vi "Micro-PL v10.0.0.vi"() -> ()   [LabVIEW 2010]
uses:
  drivers/Oxford ITC/ITCAPPS.LLB/ITCSetup.ctl
  drivers/Oxford ITC/ITCSUBS.LLB/ITCIO.ctl
  drivers/Oxford ITC/BUSGEN.LLB/OxfordAddress.ctl
  drivers/Oxford ITC/ITCSUBS.LLB/ITCVersion.ctl
  subvi/ESA-C/TypeDefs/ESA-C Live Controls.ctl
  subvi/ESA-C/TypeDefs/ESA-C Current Values.ctl
  subvi/ESA-C/TypeDefs/ESA-C Connection Settings.ctl
  subvi/ESA-C/TypeDefs/ESA-C Set Positions.ctl
  subvi/ITC503/TypeDefs/ITC503 Settings.ctl
  subvi/ITC503/TypeDefs/ITC503 Current Values.ctl
  subvi/iHR550/TypeDefs/iHR Current Values.ctl
  subvi/iHR550/TypeDefs/iHR Settings.ctl
  subvi/Mapping/TypeDefs/Mapping Spectra Params.ctl
  <vilib>/Utility/miscctls.llb/LVPointTypeDef.ctl
  drivers/Horiba Spectrum One 3000V/Lib/CCD_command.llb/Comm Params.ctl
panel:
  out "Int. Time Temp":dbl
  out "Wavelengths (nm)":dbl[](array[numeric])
  out "Measurement Running":bool
  out "ITC503s Running":bool
  out "Drive Running":bool
  out "CCD3500V Running":bool
  out "iHR550 Running":bool
  in  "Exit":bool
  out "iHR550 Status":bool
  out "Drive Status":bool
  out "CCD3500V Status":bool
  out "ITC503 Status":bool
  in  "CCD3500V Connection":T1={"Comm Interface"=1, "BUS"=0, "Address"=5, "Com Port"=0}
  out "Video Running":bool
  out "iHR550 RefNum":refnum<k7> caption="Mono RefNum out"
  out "ITC Setup":T2={"Description"="", "IO Info"={"Address"={"Com Port"=1, "ISOBUS Address"=1, "GPIB Address"=24, "Communication"=enum."ISOBUS"}, "Version"=enum."ITC503", "Ch 1 dec places"=1, "Ch 2 dec places"=1, "Ch 3 dec places"=1, "Ch1 Name"="", "Ch2 Name"="", "Ch3 Name"=""}}
  in  "Register":T6(tab)
  in  "iHR550 Force Init":bool=TRUE
  in  "iHR550 Connect":bool
  in  "iHR550 ID":string(combo)="iHR550" caption="Monochromator ID"
  out "ITC503 Current Values":T7 {"ITC503 Gradient" format="%.2f"; "ITC503 Setpoint" min=-273.0 max=300000.0 step=0.0001 format="%.1f"; "ITC503 I" format="%_1f"; "ITC503 P" format="%_1f"; "ITC503 Temperature" min=0.0 max=1645.0 step=1e-05 format="%.2f"; "ITC503 Heater" min=0.0 max=100.0 step=0.01 scale=0.0..100.0}
  in  "ITC503 Settings":T8={"ITC503 Set Setpoint"=0.0, "ITC503 Set Auto Heater"=TRUE, "ITC503 Set Auto PID"=TRUE, "P"=0.0, "I"=0.0, "D"=0.0} {"D" min=0.0 max=100.0 step=0.1 format="%.1f"; "I" min=0.0 max=100.0 step=0.1 format="%.1f"; "P" min=0.0 max=100.0 step=0.1 format="%.1f"; "ITC503 Set Setpoint" min=-273.0 max=300000.0 step=0.1 format="%.1f"}
  in  "ITC503 Configure":bool
  in  "ITC503 Connect":bool
  in  "ITC503 Selector":u16(ring) caption="Select Device" items=["ITC503s"]
  out "Drive Current Values":T9 {"Position"."Drive Z Position" min=-273.0 max=300000.0 step=0.0001 format="%.1f"; "Position"."Drive Y Position" min=-273.0 max=300000.0 step=0.0001 format="%.1f"; "Position"."Drive X Position" min=-273.0 max=300000.0 step=0.0001 format="%.1f"; "Voltages"."Drive Z Voltage" min=-273.0 max=300000.0 step=0.0001 format="%.1f"; "Voltages"."Drive Y Voltage" min=-273.0 max=300000.0 step=0.0001 format="%.1f"; "Voltages"."Drive X Voltage" min=-273.0 max=300000.0 step=0.0001 format="%.1f"}
  in  "Drive Connection":T10={"Objective GPIB-Port"=4, "Stage GPIB-Port"=4, "Drive Selector"=0, "Drive Velocity (V/s)"=5.0} {"Drive Velocity (V/s)" min=10.0 max=160.0 step=0.1 format="%.1f"; "Drive Selector" items=["Obj.", "Stage"]; "Stage GPIB-Port" min=1 max=20 step=1 format="%#.0f"; "Objective GPIB-Port" min=1 max=20 step=1 format="%#.0f"}
  in  "Drive Connect":bool
  out "CCD3500 Temperature":dbl caption="Temp. (°C)" min=10.0 max=160.0 step=0.1 format="%.1f"
  in  "CCD3500V GPIB-Port":i32=5 caption="GPIB-Port" min=1 max=20 step=1 format="%#.0f"
  in  "CCD3500V Connect":bool
  in  "CCD3000 Current Rep.":string="0/0"
  in  "Video Show":bool
  in  "Drive GoTo":bool caption="Objective Move Abs."
  in  "Drive New Positions":T11 {"Drive X Set" min=10.0 max=160.0 step=0.1 format="%.1f"; "Drive Z Set" min=10.0 max=160.0 step=0.1 format="%.1f"; "Drive Y Set" min=10.0 max=160.0 step=0.1 format="%.1f"}
  in  "Spectrum Autosave":bool=TRUE caption="iHR550 Force Init"
  in  "CCD3500 Preview":bool
  in  "CCD3500 Acquire":bool
  in  "Spectra Settings":T12={"Integration Time"=1.0, "Repetitions"=1, "Mapping Spectra"=TRUE} caption="Mapping Spectra Settings" {"Repetitions" min=1 max=100 step=1; "Integration Time" min=0.1 max=6000.0 step=0.1 format="%.1f"}
  in  "Spectrum Save":bool
  out "Spectrum":cluster{dbl[], dbl[]}(graph)
  in  "Mapping Start":bool
  in  "iHR550 Configure":bool
  in  "iHR Settings":T13={"iHR550 Set Exit Mirror"=2, "iHR550 Set Side Exit"=0.0, "iHR550 Set Front Entrance"=0.0, "iHR550 Set Wavelength"=897.9988, "iHR550 Set Grating"=0, "iHR550 Set Grating Switch"=FALSE, "iHR550 Set Wavelength Switch"=FALSE, "iHR550 Set Mirror Switch"=FALSE, "iHR550 Set Slits Switch"=FALSE} {"iHR550 Set Grating" items=["1800"=1, "600"=2, "150"=3]; "iHR550 Set Wavelength" min=0.0 max=1500.0 step=1.0; "iHR550 Set Side Exit" min=0.0 max=2000.0 step=1.0; "iHR550 Set Exit Mirror" items=["Front"=2, "Side"=3]}
  out "iHR Current Values":T14={"iHR 550 Front Entrance"=0.0, "iHR550 Side Exit"=0.0, "iHR550 Wavelength"=897.9988, "iHR550 Exit Mirror"=2, "iHR550 Grating"="1", "Grating Index"=1} {"iHR550 Exit Mirror" items=["EntranceMirror", "ExitMirror", "Front", "Side"]}
  out "Drive Live Current Values":T9 {"Position"."Drive Z Position" min=-273.0 max=300000.0 step=0.0001 format="%.1f"; "Position"."Drive Y Position" min=-273.0 max=300000.0 step=0.0001 format="%.1f"; "Position"."Drive X Position" min=-273.0 max=300000.0 step=0.0001 format="%.1f"; "Voltages"."Drive Z Voltage" min=-273.0 max=300000.0 step=0.0001 format="%.1f"; "Voltages"."Drive Y Voltage" min=-273.0 max=300000.0 step=0.0001 format="%.1f"; "Voltages"."Drive X Voltage" min=-273.0 max=300000.0 step=0.0001 format="%.1f"}
  in  "Drive Live Controls":T15={"Snapshot"=FALSE, "Move Step"=1.0, "Move Home"=FALSE, "Move Down"=FALSE, "Move Up"=FALSE, "Move Left"=FALSE, "Move Right"=FALSE, "Move Out"=FALSE, "Move In"=FALSE} {"Move Step" min=0.0 max=30.0 step=0.1 format="%.1f"}
  # "Correlation Setup"
  # "Active"
  # "Active"
  # "ITC"
  # "iHR"
  # "Drive"
  # "CCD"
  # "Status"
  # "CCD"
  # "ITC"
  # "iHR"
  # "Drive"
  # "Monochromator"
  # "Cryostat"
  # "Drives"
  # "CCD-Camera"
  # "Drive Control"
  # "CCD"
  # "Spectrum"
  # "Mapping"
  # "Launch the Spectral Mapping VI and Raman Tool Set 2.0 in a new window."
  # "Monochromator"
  # "XY"
  # "Z"
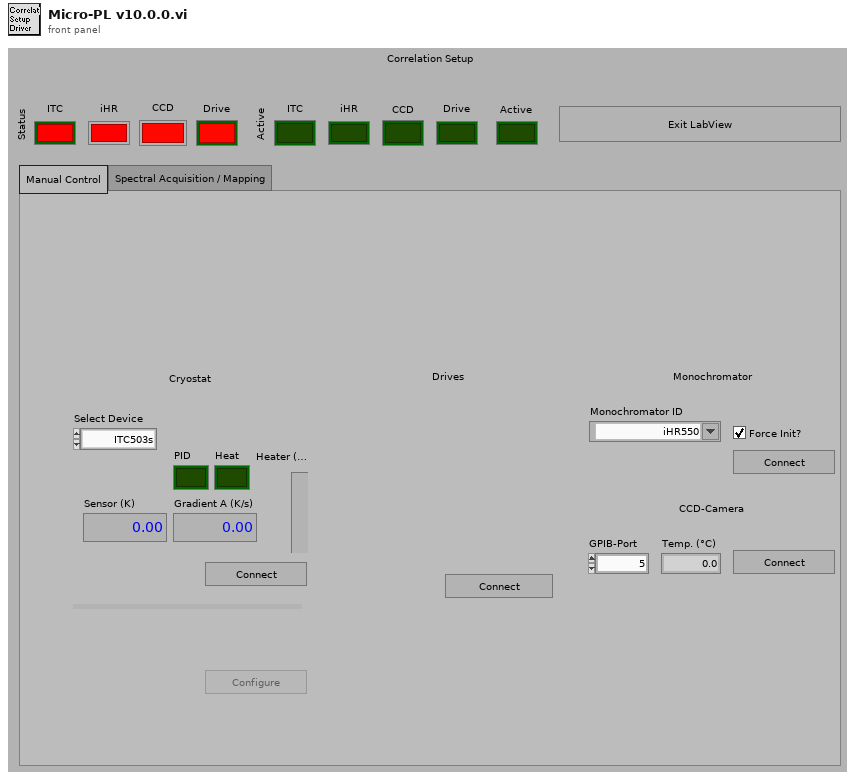
[diagram p1: front panel]
types:
  T1 = cluster{"Comm Interface":u16, "BUS":i16, "Address":i16, "Com Port":i32}
  T2 = typedef "ITCSetup.ctl" = cluster{"Description":string, "IO Info":T3}
  T3 = typedef "ITCIO.ctl" = cluster{"Address":T4, "Version":T5, "Ch 1 dec places":i16, "Ch 2 dec places":i16, "Ch 3 dec places":i16, "Ch1 Name":string, "Ch2 Name":string, "Ch3 Name":string}
  T4 = typedef "OxfordAddress.ctl" = cluster{"Com Port":i32, "ISOBUS Address":i32, "GPIB Address":i16, "Communication":enum16{"RS232", "ISOBUS", "GPIB", "Gateway"}}
  T5 = typedef "ITCVersion.ctl" = enum16{"ITC502", "ITC503", "ITC601"}
  T6 = enum32{"Manual Control", "Spectral Acquisition / Mapping"}
  T7 = typedef "ITC503 Current Values.ctl" = cluster{"ITC503 Heater":dbl, "ITC503 Temperature":dbl, "ITC503 P":dbl, "ITC503 I":dbl, "ITC503 D":dbl, "ITC503 Setpoint":dbl, "ITC503 Gradient":dbl, "ITC503 Heater Auto":bool, "ITC503 PID Auto":bool}
  T8 = typedef "ITC503 Settings.ctl" = cluster{"ITC503 Set Setpoint":dbl, "ITC503 Set Auto Heater":bool, "ITC503 Set Auto PID":bool, "P":dbl, "I":dbl, "D":dbl}
  T9 = typedef "ESA-C Current Values.ctl" = cluster{"Voltages":cluster{"Drive X Voltage":dbl, "Drive Y Voltage":dbl, "Drive Z Voltage":dbl}, "Position":cluster{"Drive X Position":dbl, "Drive Y Position":dbl, "Drive Z Position":dbl}}
  T10 = typedef "ESA-C Connection Settings.ctl" = cluster{"Objective GPIB-Port":i32, "Stage GPIB-Port":i32, "Drive Selector":u16, "Drive Velocity (V/s)":dbl}
  T11 = typedef "ESA-C Set Positions.ctl" = cluster{"Drive X Set":dbl, "Drive Y Set":dbl, "Drive Z Set":dbl}
  T12 = typedef "Mapping Spectra Params.ctl" = cluster{"Integration Time":dbl, "Repetitions":u16, "Mapping Spectra":bool}
  T13 = typedef "iHR Settings.ctl" = cluster{"iHR550 Set Exit Mirror":u16, "iHR550 Set Side Exit":dbl, "iHR550 Set Front Entrance":dbl, "iHR550 Set Wavelength":dbl, "iHR550 Set Grating":u16, "iHR550 Set Grating Switch":bool, "iHR550 Set Wavelength Switch":bool, "iHR550 Set Mirror Switch":bool, "iHR550 Set Slits Switch":bool}
  T14 = typedef "iHR Current Values.ctl" = cluster{"iHR 550 Front Entrance":dbl, "iHR550 Side Exit":dbl, "iHR550 Wavelength":dbl, "iHR550 Exit Mirror":i32, "iHR550 Grating":string, "Grating Index":i32}
  T15 = typedef "ESA-C Live Controls.ctl" = cluster{"Snapshot":bool, "Move Step":dbl, "Move Home":bool, "Move Down":bool, "Move Up":bool, "Move Left":bool, "Move Right":bool, "Move Out":bool, "Move In":bool}
  T16 = typedef "LVPointTypeDef.ctl" = cluster{"Horizontal":i16, "Vertical":i16}
  T17 = enum16{"CCD Temperature Z345", "CCD Temperature Z308", "CCD Gain"}
  T18 = enum8{"Enabled", "Disabled", "Disabled and Grayed Out"}
  T19 = typedef "Comm Params.ctl" = cluster{"Comm Interface":u16, "BUS":i16, "Address":i16, "Com Port":i32}
  T20 = cluster{"CCD3000 Connection":T19, "Drive Connection Settings":T10, "ITC503 Current Values":T7, "Wavelengths (nm)":dbl[], "Drive Current Values":T9, "iHR Current Values":T14, "Spectra Settings":T12, "CCD3500 Temperature":dbl}
  T21 = cluster{"Intensities":dbl[], "Wavelengths":dbl[]}
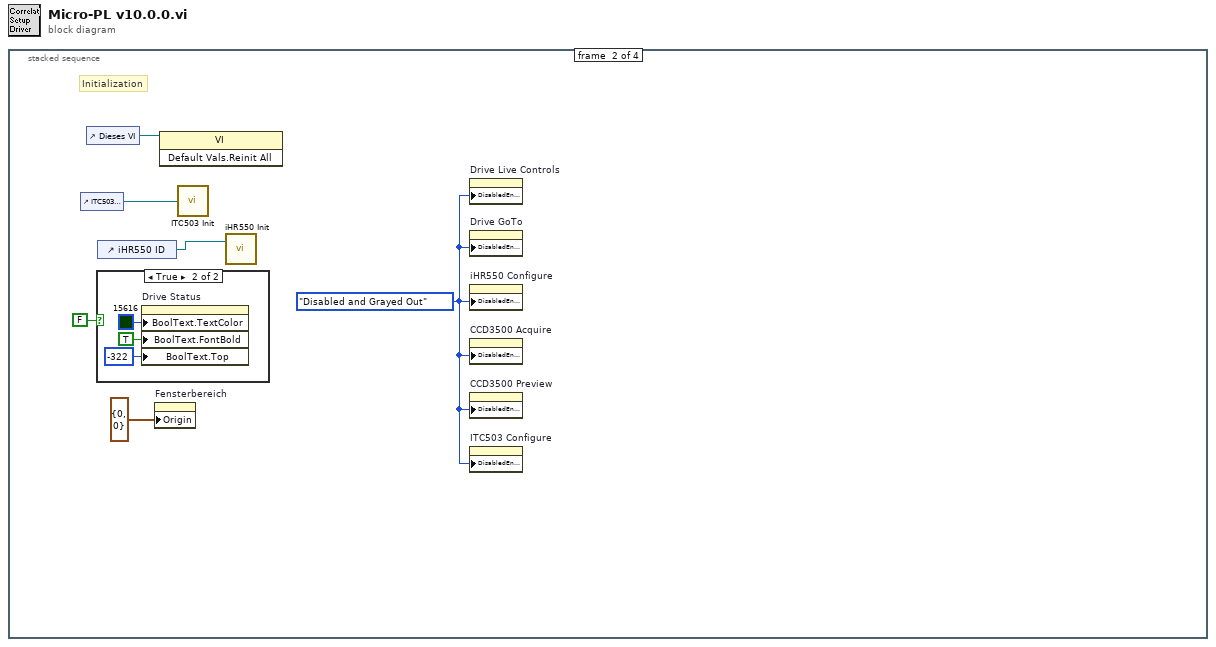
[diagram p0: block diagram]
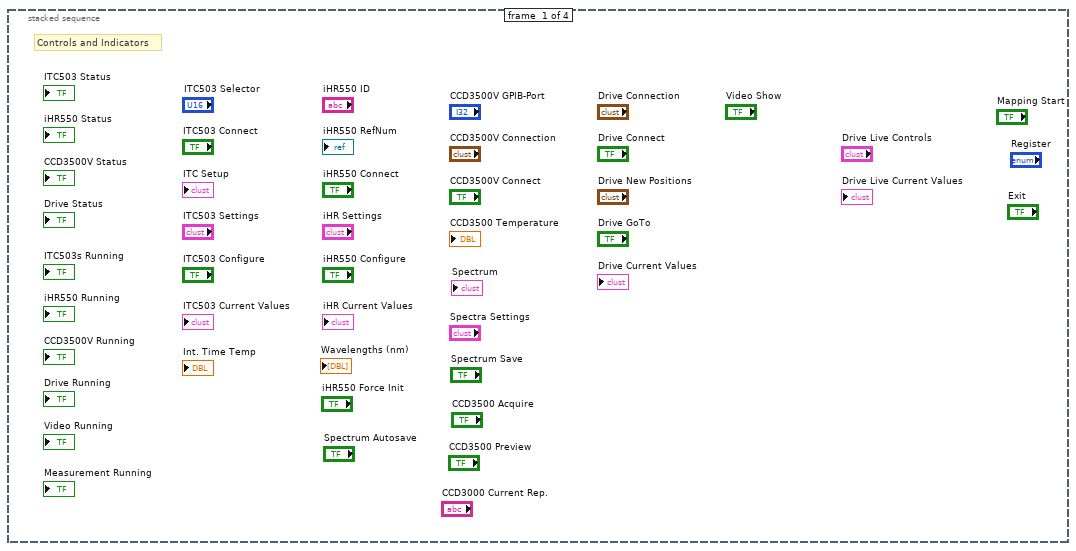
[diagram p2: hidden frame]
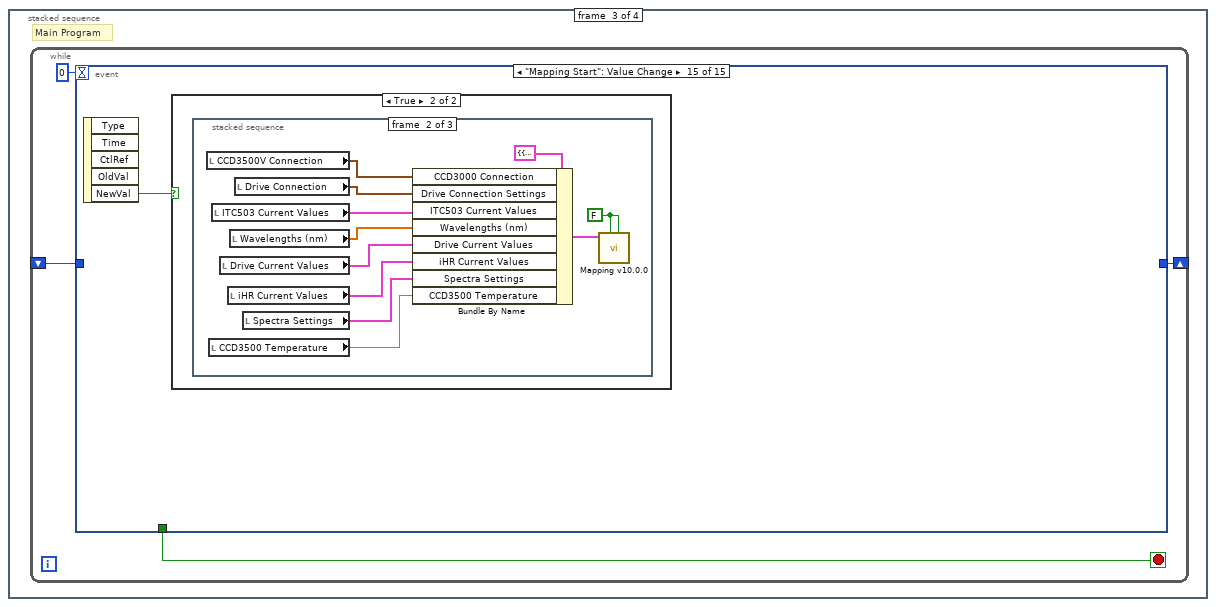
[diagram p4: hidden frame]
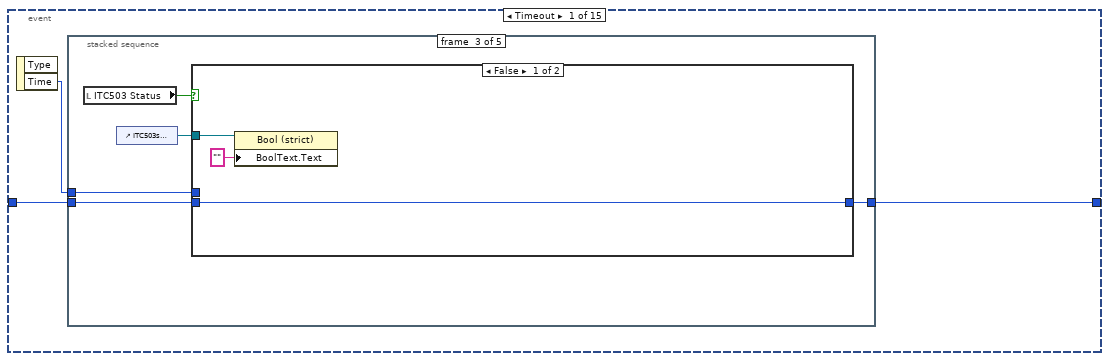
[diagram p5: hidden frame]
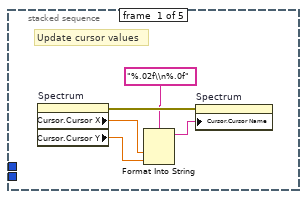
[diagram p6: hidden frame]
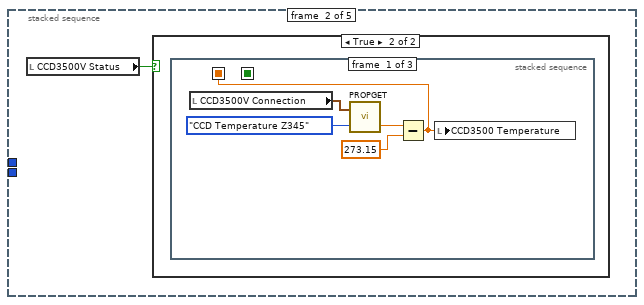
[diagram p7: hidden frame]
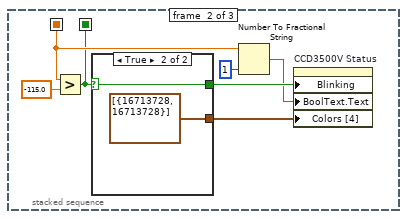
[diagram p9: hidden frame]
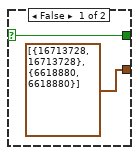
[diagram p10: hidden frame]
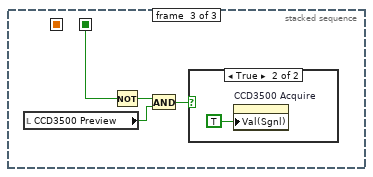
[diagram p11: hidden frame]
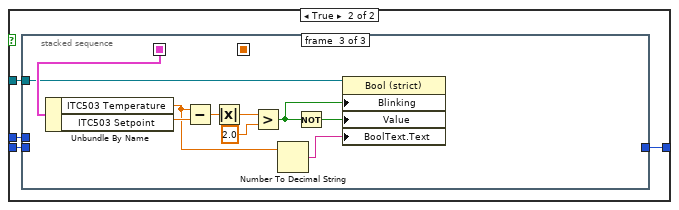
[diagram p13: hidden frame]
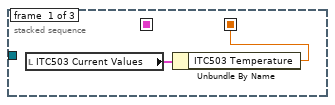
[diagram p14: hidden frame]
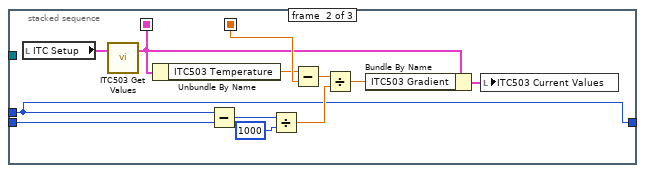
[diagram p15: hidden frame]
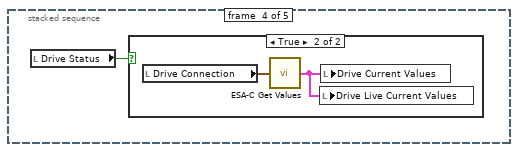
[diagram p16: hidden frame]
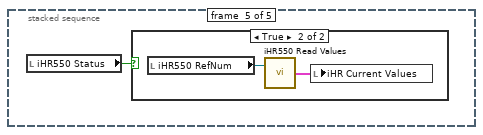
[diagram p18: hidden frame]
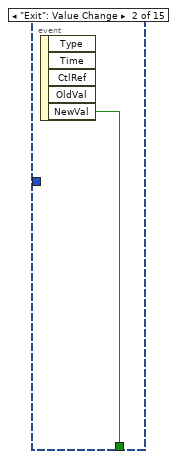
[diagram p20: hidden frame]
diagram:
  n1 = stacked-sequence {
    frame #0 {
      # "Controls and Indicators"
    }
    frame #1 {
      w1 = T18."Disabled and Grayed Out" ("Deaktiviert")
      # "Initialization"
      n2 = control-ref of="ITC503 Selector"() -> (w6:refnum<vi>)
      n3 = control-ref of="Dieses VI"() -> (w5:refnum<vi>)
      n4 = case shown="True" FALSE {
        frame False {
        }
        frame True {
          n5 = property on="Drive Status" class="Bool (strict)"("BoolText.TextColor"=u32 15616, "BoolText.FontBold"=TRUE ("Boolescher Text.Schriftart:Fett"), "BoolText.Top"=-322 ("Boolescher Text.Position:Oben")) -> ()  [unwired: 2 in, 2 out]
        }
      }
      n6 = control-ref of="iHR550 ID"() -> (w4:refnum<vi>)
      n7 = property on="Fensterbereich" class="Pane"("Origin"=T16 {"Horizontal"=0, "Vertical"=0}) -> ()  [unwired: 2 in, 2 out]
      n8 = invoke class="VI" method="Default Vals.Reinit All"(reference=w5) -> ()  [unwired: 2 in, 3 out]
      n9 = call "ITC503 Init.vi"("ITC Selector"=w6) -> ()  [unwired: 1 in]
      n10 = call "iHR550 Init.vi"("Mono ID"=w4) -> ()  [unwired: 2 in]
      n11 = property on="Drive Live Controls" class="Clust (strict)"("DisabledEnum"=w1) -> ()  [unwired: 2 in, 2 out]
      n12 = property on="Drive GoTo" class="Bool (strict)"("DisabledEnum"=w1) -> ()  [unwired: 2 in, 2 out]
      n13 = property on="iHR550 Configure" class="Bool (strict)"("DisabledEnum"=w1) -> ()  [unwired: 2 in, 2 out]
      n14 = property on="CCD3500 Acquire" class="Bool (strict)"("DisabledEnum"=w1) -> ()  [unwired: 2 in, 2 out]
      n15 = property on="CCD3500 Preview" class="Bool (strict)"("DisabledEnum"=w1) -> ()  [unwired: 2 in, 2 out]
      n16 = property on="ITC503 Configure" class="Bool (strict)"("DisabledEnum"=w1) -> ()  [unwired: 2 in, 2 out]
    }
    frame #2 {
      # "Main Program"
      n17 = while "Main-Program" {
        shift-right: [w11] -> _
        shift-left: _ -> [w10]
        stop <- w13 stop-if-true
        n18 = event shown="[14] \"Mapping Start\": Value Change" {
          selector: _ -> [_ _ _ _ _ _ _ _ _ _ _ _ _ _ _]
          dyn-events: _ -> [_ _ _ _ _ _ _ _ _ _ _ _ _ _ _]
          timeout: 0 -> [_ _ _ _ _ _ _ _ _ _ _ _ _ _ _]
          tunnel: [_ w86 _ _ _ _ _ _ _ _ _ _ _ _ _] -> w13
          tunnel: w10 -> [w15 _ _ _ _ _ _ _ _ _ _ _ _ _ _]
          tunnel: [w14 _ _ _ _ _ _ _ _ _ _ _ _ _ _] -> w11
          event Timeout {
            n19 = event-data() -> ("Time"=w16:u32)  [unwired: 1 in, 1 out]
            n20 = stacked-sequence {
              tunnel: w16 -> [_ _ w47 _ _]
              tunnel: w15 -> [_ _ w46 _ _]
              tunnel: [_ _ w45 _ _] -> w14
              frame #0 {
                # "Update cursor values"
                n21 = property on="Spectrum" class="XYGraph (strict)"() -> (error out=w21:errorcluster, "Cursor.Cursor X"=w20:dbl, "Cursor.Cursor Y"=w19:dbl)  [unwired: 2 in, 1 out]
                n22 = Format Into String(format string="%.02f\\n%.0f", w20, w19) -> (resulting string=w17:string)  [unwired: 2 in, 1 out]
                n23 = property on="Spectrum" class="XYGraph (strict)"(error in=w21, "Cursor.Cursor Name"=w17) -> ()  [unwired: 1 in, 2 out]
              }
              frame #1 {
                n24 = local read "CCD3500V Status"() -> (w22:bool)
                n25 = case shown="True" w22 {
                  frame False {
                  }
                  frame True {
                    n26 = stacked-sequence {
                      seq-local: [w23 _ _] -> [_ w32 _]
                      seq-local: [_ w28 _] -> [_ _ w42]
                      frame #0 {
                        n27 = local read "CCD3500V Connection"() -> (w27:T1)
                        n28 = call "PROPGET.VI"("CCD Prop ID"=T17."CCD Temperature Z345", "Comm Params"=w27) -> ("Output Param"=w25:dbl)  [unwired: 1 out]
                        n29 = Subtract(x=w25, y=273.15) -> (x-y=w23:dbl)
                        n30 = local write "CCD3500 Temperature"(w23) -> ()
                      }
                      frame #1 {
                        n31 = Greater?(x=w32, y=-115.0) -> (0:w28:bool)
                        n32 = case shown="True" w28 {
                          selector: w28 -> [w36 w38]
                          tunnel: [cluster{u32, u32}[] [{16713728, 16713728}, {6618880, 6618880}] ("Farben [4]") cluster{u32, u32}[] [{16713728, 16713728}] ("Farben [4]")] -> w29
                          tunnel: [w36 w38] -> w31
                          frame False {
                          }
                          frame True {
                          }
                        }
                        n33 = Number To Fractional String(number=w32, precision (6)=i16 1 ("Genauigkeit (6)")) -> (F-format string=w30:string)  [unwired: 2 in]
                        n34 = property on="CCD3500V Status" class="Bool (strict)"("Blinking"=w31, "BoolText.Text"=w30, "Colors [4]"=w29) -> ()  [unwired: 2 in, 2 out]
                      }
                      frame #2 {
                        n35 = local read "CCD3500 Preview"() -> (w40:bool)
                        n36 = Not(x=w42) -> (.not. x?=w41:bool)
                        n37 = And(x=w41, y=w40) -> (x .and. y?=w39:bool)
                        n38 = case shown="True" w39 {
                          frame False {
                          }
                          frame True {
                            n39 = property on="CCD3500 Acquire" class="Bool (strict)"("Val(Sgnl)"=TRUE ("Wert (signalisierend)")) -> ()  [unwired: 2 in, 2 out]
                          }
                        }
                      }
                    }
                  }
                }
              }
              frame #2 {
                n40 = local read "ITC503 Status"() -> (w48:bool)
                n41 = control-ref of="ITC503s Running"() -> (w44:refnum<vi>)
                n42 = case shown="False" w48 {
                  tunnel: w47 -> [_ w55]
                  tunnel: w46 -> [w51 w54]
                  tunnel: [w51 w53] -> w45
                  tunnel: w44 -> [w50 w52]
                  frame False {
                    n43 = property class="Bool (strict)"(reference=w50, "BoolText.Text"="" ("Boolescher Text.Text")) -> ()  [unwired: 1 in, 2 out]
                  }
                  frame True {
                    n44 = stacked-sequence {
                      seq-local: [_ w66 _] -> [_ _ w75]
                      seq-local: [w56 _ _] -> [_ w67 _]
                      tunnel: w55 -> [_ w58 _]
                      tunnel: w54 -> [_ w61 _]
                      tunnel: [_ w58 _] -> w53
                      tunnel: w52 -> [_ _ w70]
                      frame #0 {
                        n45 = local read "ITC503 Current Values"() -> (w57:T7)
                        n46 = Unbundle By Name(w57) -> ("ITC503 Temperature"=w56:dbl)
                      }
                      frame #1 {
                        n47 = local read "ITC Setup"() -> (w69:T2)
                        n48 = call "ITC503 Get Values.vi"("ITC Setup"=w69) -> ("ITC503 Current Values"=w66:T7)  [unwired: 1 in, 1 out]
                        n49 = Unbundle By Name(w66) -> ("ITC503 Temperature"=w65:dbl)
                        n50 = Subtract(x=w58, y=w61) -> (x-y=w63:u32)
                        n51 = Divide(x=w63, y=u32 1000) -> (x/y=w62:dbl)
                        n52 = Subtract(x=w65, y=w67) -> (x-y=w60:dbl)
                        n53 = Divide(x=w60, y=w62) -> (x/y=w59:dbl)
                        n54 = Bundle By Name(cluster=w66, "ITC503 Gradient"=w59) -> (w68:T7)
                        n55 = local write "ITC503 Current Values"(w68) -> ()
                      }
                      frame #2 {
                        n56 = Unbundle By Name(w75) -> ("ITC503 Temperature"=w71:dbl, "ITC503 Setpoint"=w76:dbl)
                        n57 = Subtract(x=w71, y=w76) -> (x-y=w77:dbl)
                        n58 = Absolute Value(x=w77) -> (abs(x)=w78:dbl)
                        n59 = Greater?(x=w78, y=2.0) -> (0:w74:bool)
                        n60 = Number To Decimal String(number=w71) -> (decimal integer string=w72:string)  [unwired: 1 in]
                        n61 = Not(x=w74) -> (.not. x?=w73:bool)
                        n62 = property class="Bool (strict)"(reference=w70, "Blinking"=w74, "Value"=w73, "BoolText.Text"=w72) -> ()  [unwired: 1 in, 2 out]
                      }
                    }
                  }
                }
              }
              frame #3 {
                n63 = local read "Drive Status"() -> (w80:bool)
                n64 = case shown="True" w80 {
                  frame False {
                  }
                  frame True {
                    n65 = local read "Drive Connection"() -> (w81:T10)
                    n66 = call "ESA-C Get Values.vi"("Drive Connection Settings"=w81) -> ("Drive Current Values"=w82:T9)
                    n67 = local write "Drive Live Current Values"(w82) -> ()
                    n68 = local write "Drive Current Values"(w82) -> ()
                  }
                }
              }
              frame #4 {
                n69 = local read "iHR550 Status"() -> (w83:bool)
                n70 = case shown="True" w83 {
                  frame False {
                  }
                  frame True {
                    n71 = local read "iHR550 RefNum"() -> (w85:refnum<k7>)
                    n72 = call "iHR550 Read Values.vi"("JYMONOLib.IJYMonoReqd"=w85) -> ("iHR Current Values"=w84:T14)  [unwired: 1 in]
                    n73 = local write "iHR Current Values"(w84) -> ()
                  }
                }
              }
            }
          }
          event "Exit": Value Change {
            n74 = event-data() -> ("NewVal"=w86:bool)  [unwired: 1 in, 4 out]
          }
          event "ITC503 Connect": Value Change {
            n75 = event-data() -> ("NewVal"=w87:bool)  [unwired: 1 in, 4 out]
            n76 = stacked-sequence {
              tunnel: w87 -> [_ w89 _]
              frame #0 {
                n77 = property on="ITC503s Running" class="Bool (strict)"("Blinking"=TRUE ("Blinkend")) -> ()  [unwired: 2 in, 2 out]
              }
              frame #1 {
                n78 = case shown="True" w89 {
                  selector: w89 -> [w94 _]
                  tunnel: [w94 w101] -> w91
                  frame False {
                    # "disconnect"
                    n79 = control-ref of="ITC503s Running"() -> (w95:refnum<vi>)
                    n80 = property class="Bool (strict)"(reference=w95, "Blinking"=w94, "Value"=w94) -> ()  [unwired: 1 in, 2 out]
                  }
                  frame True {
                    # "connect"
                    n81 = local read "ITC503 Selector"() -> (w102:u16)
                    n82 = call "ITC503 Connect.vi"("ITC Selector"=w102) -> ("ITC Setup"=w100:T2, "Connected"=w101:bool)
                    n83 = local write "ITC Setup"(w100) -> ()
                    n84 = call "ITC503 Get Values.vi"("ITC Setup"=w100) -> ("ITC503 Current Values"=w99:T7)  [unwired: 1 in, 1 out]
                    n85 = Unbundle By Name(w99) -> ("ITC503 Setpoint"=w96:dbl)
                    n86 = Bundle By Name(cluster=T8 {"ITC503 Set Setpoint"=0.0, "ITC503 Set Auto Heater"=TRUE, "ITC503 Set Auto PID"=TRUE, "P"=0.0, "I"=0.0, "D"=0.0} ("ITC503 Settings"), "ITC503 Set Setpoint"=w96) -> (w97:T8)
                    n87 = local write "ITC503 Settings"(w97) -> ()
                  }
                }
                n88 = case shown="False" w91 {
                  tunnel: [T18."Disabled and Grayed Out" ("Deaktiviert") T18."Enabled" ("Deaktiviert")] -> w90
                  frame False {
                  }
                  frame True {
                  }
                }
                n89 = local write "ITC503 Status"(w91) -> ()
                n90 = local write "ITC503 Connect"(w91) -> ()
                n91 = property on="ITC503 Configure" class="Bool (strict)"("DisabledEnum"=w90) -> ()  [unwired: 2 in, 2 out]
              }
              frame #2 {
                n92 = property on="ITC503s Running" class="Bool (strict)"("Blinking"=FALSE ("Blinkend")) -> ()  [unwired: 2 in, 2 out]
              }
            }
          }
          event "iHR550 Connect": Value Change {
            n93 = event-data() -> ("NewVal"=w104:bool)  [unwired: 1 in, 4 out]
            n94 = stacked-sequence {
              tunnel: w104 -> [_ w107 _]
              frame #0 {
                n95 = property on="iHR550 Running" class="Bool (strict)"("Blinking"=TRUE ("Blinkend")) -> ()  [unwired: 2 in, 2 out]
              }
              frame #1 {
                n96 = case shown="True" w107 {
                  selector: w107 -> [w111 _]
                  tunnel: [w111 w124] -> w106
                  frame False {
                    # "disconnect"
                  }
                  frame True {
                    # "connect"
                    n97 = local read "iHR550 Force Init"() -> (w122:bool)
                    n98 = control-ref of="iHR550 Set Grating"() -> (w123:refnum<vi>)
                    n99 = local read "iHR550 ID"() -> (w125:string)
                    n100 = call "iHR550 Connect.vi"("Force\nInitialization"=w122, "Grating Selector"=w123, "Mono ID"=w125) -> ("Initialized"=w124:bool, "iHR550 RefNum"=w121:refnum<k7>)  [unwired: 2 in, 4 out]
                    n101 = local write "iHR550 RefNum"(w121) -> ()
                    n102 = call "iHR550 Read Values.vi"("JYMONOLib.IJYMonoReqd"=w121) -> ("iHR Current Values"=w113:T14)  [unwired: 1 in]
                    n103 = local write "iHR Current Values"(w113) -> ()
                    n104 = Unbundle By Name(w113) -> ("iHR 550 Front Entrance"=w119:dbl, "iHR550 Side Exit"=w118:dbl, "iHR550 Wavelength"=w117:dbl, "iHR550 Exit Mirror"=w116:i32, "Grating Index"=w114:i32)
                    n105 = call "iHR550 Convert Axis.vi"("iHR Current Values"=w113) -> ("Wavelengths (nm)"=w112:dbl[])
                    n106 = local write "Wavelengths (nm)"(w112) -> ()
                    n107 = Bundle By Name(cluster=T13 {"iHR550 Set Exit Mirror"=0, "iHR550 Set Side Exit"=0.0, "iHR550 Set Front Entrance"=0.0, "iHR550 Set Wavelength"=0.0, "iHR550 Set Grating"=0, "iHR550 Set Grating Switch"=FALSE, "iHR550 Set Wavelength Switch"=FALSE, "iHR550 Set Mirror Switch"=FALSE, "iHR550 Set Slits Switch"=FALSE} ("iHR Settings"), "iHR550 Set Front Entrance"=w119, "iHR550 Set Side Exit"=w118, "iHR550 Set Wavelength"=w117, "iHR550 Set Exit Mirror"=w116, "iHR550 Set Grating"=w114) -> (w115:T13)
                    n108 = local write "iHR Settings"(w115) -> ()
                  }
                }
                n109 = local write "iHR550 Status"(w106) -> ()
                n110 = local write "iHR550 Connect"(w106) -> ()
                n111 = case shown="False" w106 {
                  tunnel: [T18."Disabled and Grayed Out" ("Deaktiviert") T18."Enabled" ("Deaktiviert")] -> w108
                  frame False {
                  }
                  frame True {
                  }
                }
                n112 = property on="iHR550 Configure" class="Bool (strict)"("DisabledEnum"=w108) -> ()  [unwired: 2 in, 2 out]
              }
              frame #2 {
                n113 = property on="iHR550 Running" class="Bool (strict)"("Blinking"=FALSE ("Blinkend")) -> ()  [unwired: 2 in, 2 out]
                n114 = local write "iHR550 Force Init"(FALSE ("iHR550 Force Init")) -> ()
              }
            }
          }
          event "CCD3500V Connect": Value Change {
            n115 = event-data() -> ("NewVal"=w128:bool)  [unwired: 1 in, 4 out]
            n116 = stacked-sequence {
              tunnel: w128 -> [_ w130 _]
              frame #0 {
                n117 = property on="CCD3500V Running" class="Bool (strict)"("Blinking"=TRUE ("Blinkend")) -> ()  [unwired: 2 in, 2 out]
              }
              frame #1 {
                n118 = case shown="True" w130 {
                  selector: w130 -> [w136 _]
                  tunnel: [w136 w137] -> w132
                  frame False {
                    # "disconnect"
                    n119 = local read "CCD3500V Connection"() -> (w135:T1)
                    n120 = call "CCDSTOP.VI"("Comm Params"=w135) -> ()  [unwired: 1 out]
                  }
                  frame True {
                    # "connect"
                    n121 = stacked-sequence {
                      seq-local: [_ w141 _] -> [_ _ w143]
                      tunnel: [_ w142 _] -> w137
                      frame #0 {
                        n122 = local read "CCD3500V GPIB-Port"() -> (w139:i32)
                        n123 = Bundle By Name(cluster=T19 {"Comm Interface"=1, "BUS"=0, "Address"=5, "Com Port"=1} ("Comm Params"), "Address"=w139) -> (w140:T19)
                        n124 = local write "CCD3500V Connection"(w140) -> ()
                      }
                      frame #1 {
                        n125 = local read "CCD3500V Connection"() -> (w141:T1)
                        n126 = call "CCD3000 Initialize.vi"("Comm Params"=w141) -> ("Success"=w142:bool)  [unwired: 9 in, 1 out]
                      }
                      frame #2 {
                        n127 = local read "Spectra Settings"() -> (w144:T12)
                        n128 = Unbundle By Name(w144) -> ("Integration Time"=w145:dbl)
                        n129 = local write "Int. Time Temp"(w145) -> ()
                        n130 = call "CCD3000 Prepare Acquisition.vi"("Mapping Spectra Settings"=w144, "Comm Params"=w143) -> ()  [unwired: 4 in]
                      }
                    }
                  }
                }
                n131 = local write "CCD3500V Connect"(w132) -> ()
                n132 = local write "CCD3500V Status"(w132) -> ()
                n133 = case shown="False" w132 {
                  tunnel: [T18."Disabled and Grayed Out" ("Deaktiviert") T18."Enabled" ("Deaktiviert")] -> w131
                  frame False {
                  }
                  frame True {
                  }
                }
                n134 = property on="CCD3500V Status" class="Bool (strict)"("BoolText.Visible"=w132) -> ()  [unwired: 2 in, 2 out]
                n135 = property on="CCD3500 Acquire" class="Bool (strict)"("DisabledEnum"=w131) -> ()  [unwired: 2 in, 2 out]
                n136 = property on="CCD3500 Preview" class="Bool (strict)"("DisabledEnum"=w131) -> ()  [unwired: 2 in, 2 out]
              }
              frame #2 {
                n137 = property on="CCD3500V Running" class="Bool (strict)"("Blinking"=FALSE ("Blinkend")) -> ()  [unwired: 2 in, 2 out]
              }
            }
          }
          event "Drive Connect": Value Change {
            n138 = event-data() -> ("NewVal"=w147:bool)  [unwired: 1 in, 4 out]
            n139 = stacked-sequence {
              tunnel: w147 -> [_ w151 _]
              frame #0 {
                n140 = property on="Drive Running" class="Bool (strict)"("Blinking"=TRUE ("Blinkend")) -> ()  [unwired: 2 in, 2 out]
              }
              frame #1 {
                n141 = local read "Drive Connection"() -> (w152:T10)
                n142 = Not(x=w151) -> (.not. x?=w153:bool)
                n143 = call "ESA-C Connect.vi"("Remote=F /Local=T"=w153, "Drive Connection Settings"=w152) -> ("Success"=w154:bool)  [unwired: 2 in]
                n144 = Exclusive Or(1:w153, 2:w154) -> (0:w155:bool)
                n145 = local write "Drive Connect"(w155) -> ()
                n146 = local write "Drive Status"(w155) -> ()
                n147 = case shown="False" w155 {
                  tunnel: [T18."Disabled and Grayed Out" ("Deaktiviert") T18."Enabled" ("Deaktiviert")] -> w150
                  tunnel: ["" ("Boolescher Text.Text") w158] -> w149
                  frame False {
                  }
                  frame True {
                    n148 = property on="Drive Selector" class="Ring (strict)"() -> ("RingText.Text"=w158:string)  [unwired: 2 in, 2 out]
                  }
                }
                n149 = property on="Drive Live Controls" class="Clust (strict)"("DisabledEnum"=w150) -> ()  [unwired: 2 in, 2 out]
                n150 = property on="Drive Status" class="Bool (strict)"("BoolText.Text"=w149) -> ()  [unwired: 2 in, 2 out]
                n151 = property on="Drive GoTo" class="Bool (strict)"("DisabledEnum"=w150) -> ()  [unwired: 2 in, 2 out]
              }
              frame #2 {
                n152 = property on="Drive Running" class="Bool (strict)"("Blinking"=FALSE ("Blinkend")) -> ()  [unwired: 2 in, 2 out]
              }
            }
          }
          event "Video Show": Value Change {
            n153 = event-data() -> ("NewVal"=w161:bool)  [unwired: 1 in, 4 out]
            n154 = case shown="False" w161 {
              frame False {
                n155 = call "Video Close.vi"() -> ()  [unwired: 11 in, 1 out]
              }
              frame True {
                n156 = call "Video Open.vi"() -> ()  [unwired: 11 in, 1 out]
              }
            }
          }
          event "ITC503 Configure": Value Change {
            n157 = event-data() -> ("NewVal"=w162:bool)  [unwired: 1 in, 4 out]
            n158 = stacked-sequence {
              tunnel: w162 -> [_ w164 _]
              frame #0 {
                n159 = property on="ITC503s Running" class="Bool (strict)"("Blinking"=TRUE ("Blinkend")) -> ()  [unwired: 2 in, 2 out]
              }
              frame #1 {
                n160 = local read "ITC503 Status"() -> (w166:bool)
                n161 = And(x=w166, y=w164) -> (x .and. y?=w165:bool)
                n162 = case shown="True" w165 {
                  frame False {
                  }
                  frame True {
                    n163 = local read "ITC503 Settings"() -> (w167:T8)
                    n164 = local read "ITC Setup"() -> (w168:T2)
                    n165 = call "ITC503 Set Values.vi"("Set Channel"=i16 1, "ITC503 Settings"=w167, "ITC Setup"=w168) -> ()  [unwired: 2 in]
                  }
                }
              }
              frame #2 {
                w170 = FALSE ("Blinkend")
                n166 = local write "ITC503 Configure"(w170) -> ()
                n167 = property on="ITC503s Running" class="Bool (strict)"("Blinking"=w170) -> ()  [unwired: 2 in, 2 out]
              }
            }
          }
          event "iHR550 Configure": Value Change {
            n168 = event-data() -> ("NewVal"=w171:bool)  [unwired: 1 in, 4 out]
            n169 = stacked-sequence {
              tunnel: w171 -> [_ w173 _]
              frame #0 {
                n170 = property on="iHR550 Running" class="Bool (strict)"("Blinking"=TRUE ("Blinkend")) -> ()  [unwired: 2 in, 2 out]
              }
              frame #1 {
                n171 = local read "iHR550 Status"() -> (w175:bool)
                n172 = local read "iHR550 RefNum"() -> (w176:refnum<k7>)
                n173 = And(x=w175, y=w173) -> (x .and. y?=w174:bool)
                n174 = case shown="True" w174 {
                  tunnel: w176 -> [_ w177]
                  frame False {
                  }
                  frame True {
                    n175 = stacked-sequence {
                      seq-local: [_ w182 _] -> [_ _ w185]
                      tunnel: w177 -> [w178 w183 _]
                      frame #0 {
                        w181 = u16 2 items=["Front"=2, "Side"=3] ("Entrance Mirror")
                        n176 = local read "iHR Settings"() -> (w179:T13)
                        n177 = call "iHR550 Set Values.vi"("Refnum out"=w178, "Entrance Mirror"=w181, "Target\nSide Entrance"=0.0 ("Target\nSide Entrance"), "iHR Settings"=w179) -> ()  [unwired: 11 in, 1 out]
                      }
                      frame #1 {
                        n178 = call "iHR550 Read Values.vi"("JYMONOLib.IJYMonoReqd"=w183) -> ("iHR Current Values"=w182:T14)  [unwired: 1 in]
                        n179 = local write "iHR Current Values"(w182) -> ()
                      }
                      frame #2 {
                        n180 = call "iHR550 Convert Axis.vi"("iHR Current Values"=w185) -> ("Wavelengths (nm)"=w184:dbl[])
                        n181 = local write "Wavelengths (nm)"(w184) -> ()
                      }
                    }
                  }
                }
              }
              frame #2 {
                w186 = FALSE ("Blinkend")
                n182 = local write "iHR550 Configure"(w186) -> ()
                n183 = property on="iHR550 Running" class="Bool (strict)"("Blinking"=w186) -> ()  [unwired: 2 in, 2 out]
              }
            }
          }
          event "CCD3500 Preview": Value Change {
            n184 = event-data() -> ("NewVal"=w187:bool)  [unwired: 1 in, 4 out]
            n185 = case shown="True" w187 {
              frame False {
              }
              frame True {
                n186 = property on="CCD3500 Acquire" class="Bool (strict)"("Val(Sgnl)"=TRUE ("Wert (signalisierend)")) -> ()  [unwired: 2 in, 2 out]
              }
            }
          }
          event "CCD3500 Acquire": Value Change {
            n187 = event-data() -> ("NewVal"=w189:bool)  [unwired: 1 in, 4 out]
            n188 = stacked-sequence {
              tunnel: w189 -> [w190 _]
              frame #0 {
                n189 = case shown="True" w190 {
                  frame False {
                  }
                  frame True {
                    n190 = local read "CCD3500V Connection"() -> (w191:T1)
                    n191 = local read "Spectra Settings"() -> (w192:T12)
                    n192 = stacked-sequence {
                      tunnel: w192 -> [w195 w207 _]
                      tunnel: w191 -> [w194 w203 _]
                      frame #0 {
                        # "prepare acquisition if settings changed"
                        n193 = Unbundle By Name(w195) -> ("Integration Time"=w193:dbl)
                        n194 = local read "Int. Time Temp"() -> (w196:dbl)
                        n195 = Equal?(x=w193, y=w196) -> (x = y?=w197:bool)
                        n196 = case shown="False" w197 {
                          tunnel: w196 -> [_ _]
                          tunnel: w195 -> [w200 _]
                          tunnel: w194 -> [w199 _]
                          tunnel: w193 -> [w198 _]
                          frame False {
                            n197 = local write "Int. Time Temp"(w198) -> ()
                            n198 = call "CCD3000 Prepare Acquisition.vi"("Mapping Spectra Settings"=w200, "Comm Params"=w199) -> ()  [unwired: 4 in]
                          }
                          frame True {
                          }
                        }
                      }
                      frame #1 {
                        n199 = local read "CCD3500 Preview"() -> (w206:bool)
                        n200 = Unbundle By Name(w207) -> ("Repetitions"=w204:u16)
                        n201 = Select(t=i8 1, s=w206, f=w204) -> (s? t:f=w202:u16)
                        n202 = for {
                          N: w202 -> [w211]
                          tunnel: w203 -> [w224]
                          shift-right: [w218] -> _
                          shift-left: u16[][] [] -> [w222]
                          i -> [w212]
                          stop <- w217 continue-if-true
                          n203 = control-ref of="CCD3500 Acquire"() -> (w216:refnum<vi>)
                          n204 = control-ref of="CCD3500V Running"() -> (w215:refnum<vi>)
                          n205 = call "CCD3000 Spectral Acquisition.vi"("Acquire"=w216, "Running"=w215, "Comm Params"=w224) -> ("Raw-Spectrum"=w223:u16[])  [unwired: 6 in, 2 out]
                          n206 = Number To Decimal String(number=w211) -> (decimal integer string=w210:string)  [unwired: 1 in]
                          n207 = Build Array (concatenate)(w223, w222) -> (w218:u16[][])
                          n208 = Increment(x=w212) -> (x+1=w208:i32)
                          n209 = Number To Decimal String(number=w208) -> (decimal integer string=w209:string)  [unwired: 1 in]
                          n210 = local read "Wavelengths (nm)"() -> (w220:dbl[])
                          n211 = Concatenate Strings(w209, "/" ("string"), w210) -> (w214:string)
                          n212 = call "CCD3000 Average Spectra.vi"("Repetitions"=w208, "Raw Spectra"=w218) -> ("Raw Spectrum"=w219:dbl[])
                          n213 = local read "CCD3500 Acquire"() -> (w217:bool)
                          n214 = local write "CCD3000 Current Rep."(w214) -> ()
                          n215 = call "CCD3000 Pixel to Wavelength v10.0.0.vi"("Wavelengths (nm)"=w220, "Raw Spectrum"=w219) -> ("Spectrum-Cluster"=w221:T21)  [unwired: 1 out]
                          n216 = local write "Spectrum"(w221) -> ()
                        }
                      }
                      frame #2 {
                        n217 = local read "Spectrum Autosave"() -> (w225:bool)
                        n218 = case shown="True" w225 {
                          frame False {
                          }
                          frame True {
                            n219 = property on="Spectrum Save" class="Bool (strict)"("Val(Sgnl)"=TRUE ("Value (Signaling)")) -> ()  [unwired: 2 in, 2 out]
                          }
                        }
                      }
                    }
                  }
                }
              }
              frame #1 {
                n220 = local write "CCD3500 Acquire"(FALSE ("Blinkend")) -> ()
                n221 = local write "CCD3000 Current Rep."("0/0" ("CCD3000 Current Rep.")) -> ()
              }
            }
          }
          event "Drive GoTo": Value Change {
            n222 = event-data() -> ("NewVal"=w229:bool)  [unwired: 1 in, 4 out]
            n223 = stacked-sequence {
              tunnel: w229 -> [_ w231 _]
              frame #0 {
                n224 = property on="Drive Running" class="Bool (strict)"("Blinking"=TRUE ("Blinkend")) -> ()  [unwired: 2 in, 2 out]
              }
              frame #1 {
                n225 = local read "Drive Status"() -> (w233:bool)
                n226 = And(x=w233, y=w231) -> (x .and. y?=w232:bool)
                n227 = case shown="True" w232 {
                  frame False {
                  }
                  frame True {
                    n228 = local read "Drive New Positions"() -> (w234:T11)
                    n229 = local read "Drive Connection"() -> (w235:T10)
                    n230 = control-ref of="Drive Running"() -> (w236:refnum<vi>)
                    n231 = call "ESA-C Move Absolute.vi"("Running"=w236, "Drive New Abs. Positions"=w234, "Drive Connection Settings"=w235) -> ()  [unwired: 2 in]
                  }
                }
              }
              frame #2 {
                w237 = FALSE ("Blinkend")
                n232 = local write "Drive GoTo"(w237) -> ()
                n233 = property on="Drive Running" class="Bool (strict)"("Blinking"=w237) -> ()  [unwired: 2 in, 2 out]
              }
            }
          }
          event Value Change {
            n234 = event-data() -> ("NewVal"=w239:bool)  [unwired: 1 in, 4 out]
            n235 = local read "Drive Status"() -> (w240:bool)
            n236 = And(x=w240, y=w239) -> (x .and. y?=w238:bool)
            n237 = case shown="True" w238 {
              frame False {
              }
              frame True {
                n238 = stacked-sequence {
                  seq-local: [w241 _] -> [_ w262]
                  frame #0 {
                    # "Move and Read"
                    n239 = flat-sequence {
                      tunnel: [w250] -> w246
                      tunnel: [w248] -> w245
                      tunnel: [w247] -> w244
                      tunnel: w246 -> [w252]
                      tunnel: w245 -> [w254]
                      tunnel: [w254] -> w243
                      tunnel: w244 -> [w253]
                      tunnel: [w251] -> w242
                      tunnel: w243 -> [w261]
                      tunnel: w242 -> [w259]
                      tunnel: [w259] -> w241
                      frame #0 {
                        n240 = local read "Drive Live Controls"() -> (w247:T15)
                        n241 = local read "Drive Connection"() -> (w248:T10)
                        n242 = control-ref of="Drive Running"() -> (w249:refnum<vi>)
                        n243 = call "ESA-C Live Control.vi"("Running"=w249, "Drive Live Controls"=w247, "Drive Connection Settings"=w248) -> ("Reset Switches"=w250:bool)  [unwired: 1 in]
                      }
                      frame #1 {
                        n244 = case shown="True" w252 {
                          tunnel: w253 -> [w255 w258]
                          tunnel: [w255 w257] -> w251
                          frame False {
                          }
                          frame True {
                            w256 = FALSE ("Move Out")
                            n245 = Bundle By Name(cluster=w258, "Move Home"=w256, "Move Down"=w256, "Move Up"=w256, "Move Left"=w256, "Move Right"=w256, "Move Out"=w256, "Move In"=w256) -> (w257:T15)
                          }
                        }
                      }
                      frame #2 {
                        n246 = local write "Drive Live Controls"(w259) -> ()
                        n247 = call "ESA-C Get Values.vi"("Drive Connection Settings"=w261) -> ("Drive Current Values"=w260:T9)
                        n248 = local write "Drive Live Current Values"(w260) -> ()
                      }
                    }
                  }
                  frame #1 {
                    # "Snapshot"
                    n249 = Unbundle By Name(w262) -> ("Snapshot"=w265:bool)
                    n250 = case shown="True" w265 {
                      selector: w265 -> [w266 _]
                      tunnel: [w266 FALSE] -> w264
                      frame False {
                      }
                      frame True {
                        n251 = call "Video Snapshot.vi"() -> ()  [unwired: 11 in, 1 out]
                      }
                    }
                    n252 = Bundle By Name(cluster=w262, "Snapshot"=w264) -> (w263:T15)
                    n253 = local write "Drive Live Controls"(w263) -> ()
                  }
                }
              }
            }
          }
          event "Spectrum Save": Value Change {
            n254 = event-data() -> ("NewVal"=w268:bool)  [unwired: 1 in, 4 out]
            n255 = stacked-sequence {
              tunnel: w268 -> [w269 _]
              frame #0 {
                n256 = case shown="True" w269 {
                  frame False {
                  }
                  frame True {
                    n257 = local read "Spectrum"() -> (w281:cluster{dbl[], dbl[]})
                    n258 = local read "CCD3500 Temperature"() -> (w273:dbl)
                    n259 = local read "ITC503 Current Values"() -> (w274:T7)
                    n260 = local read "Drive Current Values"() -> (w275:T9)
                    n261 = local read "iHR Current Values"() -> (w277:T14)
                    n262 = local read "Spectra Settings"() -> (w276:T12)
                    n263 = Unbundle(w281) -> (w280:dbl[], w279:dbl[])
                    n264 = Build Array(w280, w279) -> (w278:dbl[][])
                    n265 = call "Export_spectrumFileName.vi"("ITC503 Current Values"=w274, "iHR Current Values"=w277, "Spectra Settings"=w276, "Drive Current Values"=w275, "CCD3500 Temperature"=w273) -> ("Filename"=w272:string)
                    n266 = local read "Spectrum Autosave"() -> (w270:bool)
                    n267 = call "Export_2DtoTxt.vi"("Auto?"=w270, "Data (2D)"=w278, "Export Type"="Spectrum", "Filename"=w272) -> ()  [unwired: 2 in]
                  }
                }
              }
              frame #1 {
                n268 = local write "Spectrum Save"(FALSE ("Spectrum Save")) -> ()
              }
            }
          }
          event "Mapping Start": Value Change {
            n269 = event-data() -> ("NewVal"=w283:bool)  [unwired: 1 in, 4 out]
            n270 = case shown="True" w283 {
              frame False {
              }
              frame True {
                n271 = stacked-sequence {
                  frame #0 {
                    n272 = property on="Measurement Running" class="Bool (strict)"("Blinking"=TRUE ("Blinkend")) -> ()  [unwired: 2 in, 2 out]
                  }
                  frame #1 {
                    w285 = FALSE ("Simulate Drive")
                    n273 = local read "CCD3500V Connection"() -> (w292:T1)
                    n274 = local read "CCD3500 Temperature"() -> (w294:dbl)
                    n275 = local read "ITC503 Current Values"() -> (w289:T7)
                    n276 = local read "Drive Current Values"() -> (w287:T9)
                    n277 = local read "iHR Current Values"() -> (w288:T14)
                    n278 = local read "Wavelengths (nm)"() -> (w290:dbl[])
                    n279 = local read "Drive Connection"() -> (w291:T10)
                    n280 = local read "Spectra Settings"() -> (w293:T12)
                    n281 = Bundle By Name(cluster=T20 {"CCD3000 Connection"={"Comm Interface"=1, "BUS"=0, "Address"=5, "Com Port"=1}, "Drive Connection Settings"={"Objective GPIB-Port"=4, "Stage GPIB-Port"=4, "Drive Selector"=0, "Drive Velocity (V/s)"=5.0}, "ITC503 Current Values"={"ITC503 Heater"=0.0, "ITC503 Temperature"=0.0, "ITC503 P"=0.0, "ITC503 I"=0.0, "ITC503 D"=0.0, "ITC503 Setpoint"=0.0, "ITC503 Gradient"=0.0, "ITC503 Heater Auto"=FALSE, "ITC503 PID Auto"=FALSE}, "Wavelengths (nm)"=[], "Drive Current Values"={"Voltages"={"Drive X Voltage"=0.0, "Drive Y Voltage"=0.0, "Drive Z Voltage"=0.0}, "Position"={"Drive X Position"=0.0, "Drive Y Position"=0.0, "Drive Z Position"=0.0}}, "iHR Current Values"={"iHR 550 Front Entrance"=0.0, "iHR550 Side Exit"=0.0, "iHR550 Wavelength"=897.9988, "iHR550 Exit Mirror"=2, "iHR550 Grating"="1", "Grating Index"=1}, "Spectra Settings"={"Integration Time"=1.0, "Repetitions"=1, "Mapping Spectra"=TRUE}, "CCD3500 Temperature"=0.0} ("Input Parameters"), "CCD3000 Connection"=w292, "Drive Connection Settings"=w291, "ITC503 Current Values"=w289, "Wavelengths (nm)"=w290, "Drive Current Values"=w287, "iHR Current Values"=w288, "Spectra Settings"=w293, "CCD3500 Temperature"=w294) -> (w286:T20)
                    n282 = call "Mapping v10.0.0.vi"("Simulate Spectra"=w285, "Simulate Drive"=w285, "Input Parameters"=w286) -> ()  [unwired: 9 in]
                  }
                  frame #2 {
                    w296 = FALSE ("Mapping Start")
                    n283 = local write "Mapping Start"(w296) -> ()
                    n284 = property on="Measurement Running" class="Bool (strict)"("Blinking"=w296) -> ()  [unwired: 2 in, 2 out]
                  }
                }
              }
            }
          }
        }
      }
    }
    frame #3 {
      # "Close Connections"
      n285 = control-ref of="Dieses VI"() -> (w297:refnum<vi>)
      n286 = invoke class="VI" method="Default Vals.Reinit All"(reference=w297) -> ()  [unwired: 2 in, 3 out]
    }
  }
